vi "Edge Detect.vi"(8 "error in":errorcluster, 10 "input 2":bool, 11 "input 1":bool) -> (0 "error out":errorcluster, 3 "output":bool)   [LabVIEW 2017, in "NI_FunctionBlock Libraries.lvlib"]
uses:
  <vilib>/functionblocks/NI_FunctionBlock Libraries.lvlib
  <vilib>/ptbypt/NI_PtbyPt.lvlib
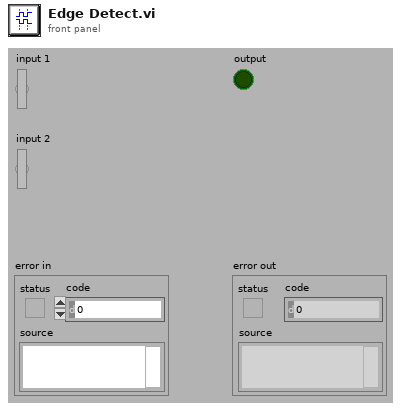
[diagram p1: front panel]
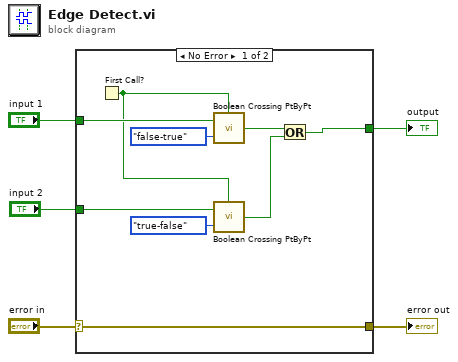
[diagram p0: block diagram]
diagram:
  n1 = case shown="No Error" "error in" {
    selector: "error in" -> [w13 w15]
    tunnel: "input 1" -> [w12 _]
    tunnel: [w6 _] -> w4
    tunnel: [w13 w15] -> w3
    tunnel: "input 2" -> [w10 _]
    frame No Error {
      n2 = First Call?() -> (First Call?: T/F=w9:bool)
      n3 = call <vilib>:"Boolean Crossing PtByPt.vi"("initialize"=w9, "direction"=enum16{"either", "false-true", "true-false"}."false-true", "input"=w12) -> ("crossing"=w7:bool)
      n4 = call <vilib>:"Boolean Crossing PtByPt.vi"("initialize"=w9, "direction"=enum16{"either", "false-true", "true-false"}."true-false", "input"=w10) -> ("crossing"=w8:bool)
      n5 = Or(x=w7, y=w8) -> (x .or. y?=w6:bool)
    }
    frame Error {
    }
  }
  "output" <- w4
  "error out" <- w3
